vi "SingleAxisMoveIncremental.vi"() -> ()   [LabVIEW 2016]
uses:
  Examples/Motion/EnableSingle.vi
  Examples/Motion/MoveIncSingle.vi
  Examples/Motion/WaitSingle.vi
  Examples/Motion/DisableSingle.vi
panel:
  out "F-format string":string
  in  "Distance":dbl
  in  "Speed":dbl
  in  "AxisName":string
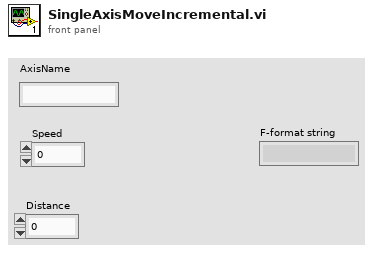
[diagram p1: front panel]
types:
  T1 = typedef "ControllerDiagPacket.ctl" = cluster{"Number of Diag Packets":i32, "Axes":T2[], "error":errorcluster}
  T2 = typedef "AxisDiagPacket.ctl" = cluster{"Axis Name":string, "Analog Input 0":dbl, "Analog Input 1":dbl, "Axis Fault (num)":i32, "Axis Fault (str)":string, "Axis Fault (bits)":cluster{"AmplifierFault":bool, "AmplifierTemperatureFault":bool, "CcwEndOfTravelLimitFault":bool, "CcwSoftwareLimitFault":bool, "CommunicationLostFault":bool, "CwEndOfTravelLimitFault":bool, "CwSoftwareLimitFault":bool, "EmergencyStopFault":bool, "EncoderFault":bool, "ExternalFault":bool, "FeedbackScalingFault":bool, "GantryMisalignFault ":bool, "HallSensorFault":bool, "InPositionTimeoutFault":bool, "MarkerSearchFault":bool, "MaxVelocityCommandFault":bool, "MissedInterruptFault":bool, "MotorTemperatureFault":bool, "None":bool, "OverCurrentFault":bool, "PositionErrorFault":bool, "PositionFeedbackFault":bool, "PowerSupplyFault":bool, "ProbeInputFault":bool, "SafeZoneFault":bool, "VelocityErrorFault":bool, "VelocityFeedbackFault":bool, "VoltageClampFault":bool}, "Axis Status (num)":i32, "Axis Status (str)":string, "Axis Status (bits)":cluster{"BacklashActive":bool, "CalibrationEnabled1D":bool, "CalibrationEnabled2D":bool, "CommandValid":bool, "DriveAbortPending":bool, "DrivePending":bool, "Enabling":bool, "GainMappingEnabled":bool, "GantryAligned":bool, "GantryRealigning":bool, "Homed":bool, "Homing":bool, "IFOVEnabled":bool, "JogGenerating":bool, "Jogging":bool, "JoystickControl":bool, "MasterSlaveControl":bool, "MotionBlocked":bool, "MotionClamped":bool, "MoveDone":bool, "None":bool, "NotVirtual":bool, "Profiling":bool, "Stability0":bool, "Stability1":bool, "TrajectoryFiltering":bool, "WaitDone":bool}, "Current Command":sgl, "Current Error":sgl, "Current Feedback":sgl, "Digital Inputs":i32, "Digital Outputs":i32, "Drive Status":i32, "Drive Status (str)":string, "Drive Status (bits)":cluster{"AccelerationPhase":bool, "AutofocusActive":bool, "BrakeOutput":bool, "CcwEndOfTravelLimitInput":bool, "CosineEncoderError":bool, "CurrentClamp":bool, "CwEndOfTravelLimitInput":bool, "DecelerationPhase":bool, "DualLoopActive":bool, "EmergencyStopInput":bool, "Enabled":bool, "EncoderClipping":bool, "GalvoCalibrationEnabled":bool, "GalvoPowerCorrection":bool, "HallAInput":bool, "HallBInput":bool, "HallCInput":bool, "HighResolutionMode":bool, "HomeLimitInput":bool, "InPosition":bool, "InPosition2":bool, "MarkerInput":bool, "MarkerLatch":bool, "MoveActive":bool, "NoMotorSupply":bool, "None":bool, "PowerLimiting":bool, "ProgrammingFlash":bool, "ProgrammingMXH":bool, "PSOHaltLatch":bool, "ServoControl":bool, "SineEncoderError":bool}, "Position Feedback Auxiliary":dbl, "Position Command":dbl, "Position Error":dbl, "Position Feedback":dbl, "Program Position Command":dbl, "Program Position Error":dbl, "Program Position Feedback":dbl, "Velocity Command":dbl, "Velocity Error":dbl, "Velocity Feedback":dbl}
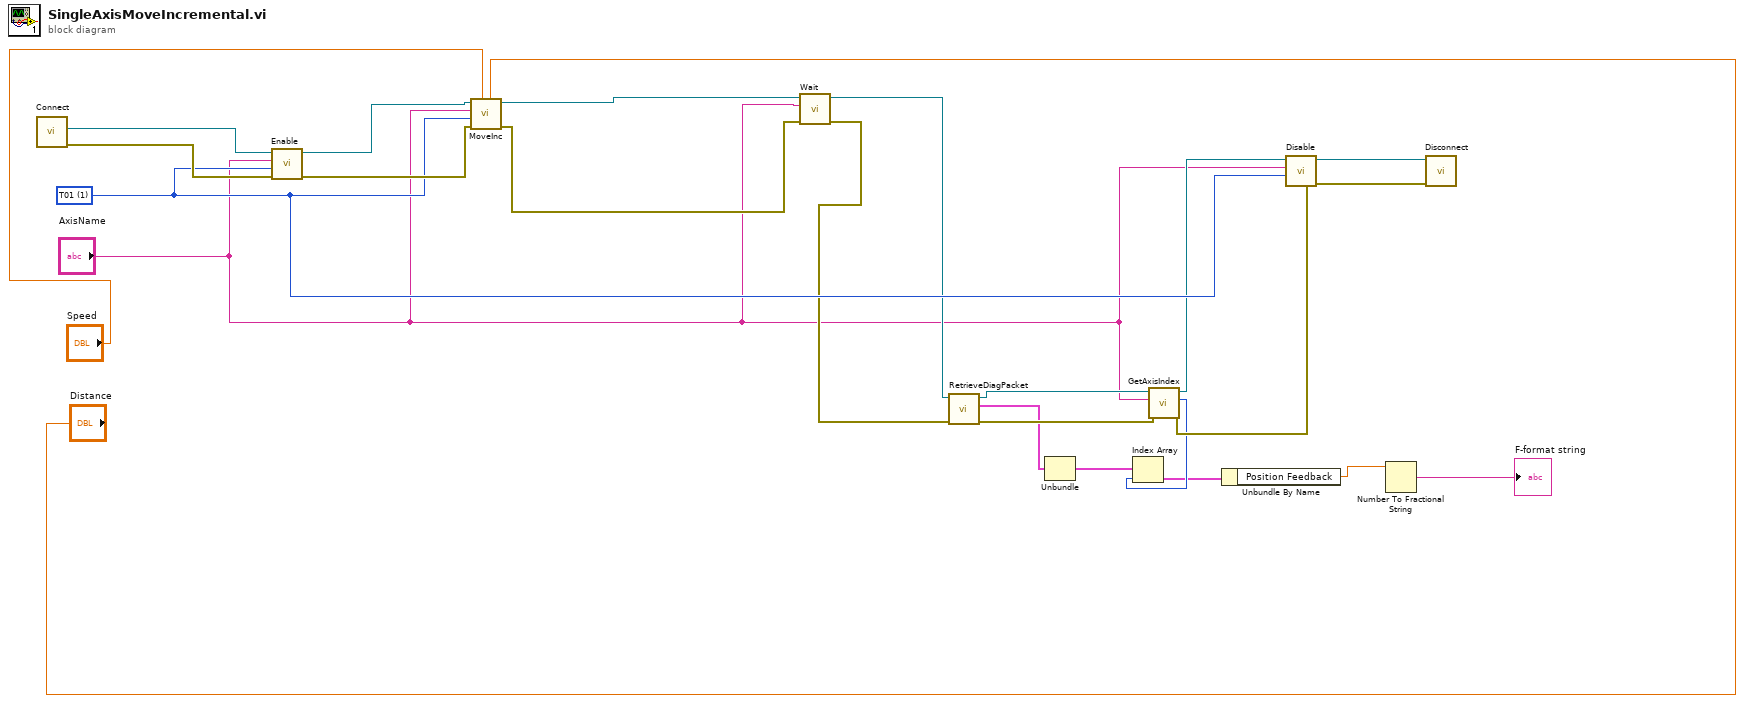
[diagram p0: block diagram]
diagram:
  w14 = 1 items=["TLibrary", "T01", "T02", "T03", "T04", "T05", "T06", "T07", "T08", "T09", "T10", "T11", "T12", "T13", "T14", "T15", "T16", "T17", "T18", "T19", "T20", "T21", "T22", "T23", "T24", "T25", "T26", "T27", "T28", "T29", "T30", "T31"] ("taskId")
  n1 = call "Connect.vi"() -> ("error out"=w23:errorcluster, "controller"=w24:refnum<k24>)  [unwired: 10 in]
  n2 = call-poly "Enable.vi"("error in (no error)"=w23, "taskId"=w14, "axis name"="AxisName", "controller in"=w24) -> ("error out"=w17:errorcluster, "controller out"=w20:refnum<k24>)  [unwired: 6 in]
  n3 = call-poly "MoveInc.vi"("distance"="Distance", "speed"="Speed", "error in (no error)"=w17, "taskId"=w14, "axis name"="AxisName", "controller in"=w20) -> ("error out"=w16:errorcluster, "controller out"=w15:refnum<k24>)  [unwired: 4 in]
  n4 = call-poly "Wait.vi"("error in (no error)"=w16, "axis name"="AxisName", "controller in"=w15) -> ("error out"=w13:errorcluster, "controller out"=w10:refnum<k24>)  [unwired: 6 in, 1 out]
  n5 = call "RetrieveDiagPacket.vi"("error in (no error)"=w13, "Controller In"=w10) -> ("error out"=w12:errorcluster, "ControllerDiagPacket"=w7:T1, "Controller Out"=w9:refnum<k24>)  [unwired: 7 in]
  n6 = Unbundle(w7) -> ("Axes"=w6:T2[])  [unwired: 2 out]
  n7 = call "GetAxisIndex.vi"("error in (no error)"=w12, "axis name"="AxisName", "controller in"=w9) -> ("error out"=w11:errorcluster, "axis index"=w5:i32, "controller out"=w8:refnum<k24>)  [unwired: 6 in]
  n8 = Index Array(array=w6, index=w5) -> (element=w3:T2)
  n9 = Unbundle By Name(w3) -> ("Position Feedback"=w2:dbl)
  n10 = call-poly "Disable.vi"("error in (no error)"=w11, "taskId"=w14, "axis name"="AxisName", "controller in"=w8) -> ("error out"=w21:errorcluster, "controller out"=w22:refnum<k24>)  [unwired: 6 in]
  n11 = Number To Fractional String(number=w2) -> (F-format string=→"F-format string":string)  [unwired: 3 in]
  n12 = call "Disconnect.vi"("error in (no error)"=w21, "controller"=w22) -> ()  [unwired: 9 in, 1 out]
